vi "I_vs_Vw_V2w_V3w(V)_MFLI_PK_v4.0_measureR_phase.vi"() -> ()   [LabVIEW 2016]
uses:
  Labview Drivers/MFLI/LabOneLabVIEW-22.02.26577/LabOneLabVIEW-22.02.26577/Zurich Instruments LabOne/Public/Data/ziTypeDemodSampleSingle.ctl
  Labview Drivers/MFLI/LabOneLabVIEW-22.02.26577/LabOneLabVIEW-22.02.26577/Zurich Instruments LabOne/Public/Configure/ziSetValueDouble.vi
  Labview Drivers/MFLI/LabOneLabVIEW-22.02.26577/LabOneLabVIEW-22.02.26577/Zurich Instruments LabOne/Public/Configure/ziGetValueDemodSampleEx.vi
  Labview Drivers/MFLI/LabOneLabVIEW-22.02.26577/LabOneLabVIEW-22.02.26577/Zurich Instruments LabOne/Zurich Instruments LabOne.lvlib
panel:
  out "I2w vs Iw":cluster{dbl, "Field Reading":dbl}[](graph)=[{2.1337108522522826e-07, "Field Reading"=1.0007121497539348e-06}, {2.0018204953851064e-08, "Field Reading"=1.0969598663661376e-07}, {3.474074033482476e-08, "Field Reading"=1.9016075130631681e-07}, {5.6400419155691035e-08, "Field Reading"=2.706780203266455e-07}, {7.134741663483111e-08, "Field Reading"=3.625194153695155e-07}, {8.711957733763268e-08, "Field Reading"=4.6186456260881066e-07}, {1.039613386460647e-07, "Field Reading"=5.541771498802743e-07}, {1.290159481540569e-07, "Field Reading"=6.517488283090827e-07}, {1.442006622421336e-07, "Field Reading"=7.441421685111633e-07}, {1.6579779771841864e-07, "Field Reading"=8.4200282004452e-07}, {1.7667431320194624e-07, "Field Reading"=9.371894272094692e-07}, {2.0346799660082097e-07, "Field Reading"=1.0346819690568719e-06}, {2.1275449478314156e-07, "Field Reading"=1.1273455634288892e-06}, {2.2792303722372882e-07, "Field Reading"=1.2246113813938451e-06}, {2.506226161778463e-07, "Field Reading"=1.3169699353558023e-06}, {2.6686786096204173e-07, "Field Reading"=1.4106741902497636e-06}, {2.979630377408132e-07, "Field Reading"=1.5068897992871093e-06}, {3.1162936250255217e-07, "Field Reading"=1.6013785409354697e-06}, {3.2854904168138843e-07, "Field Reading"=1.7007967107121696e-06}, {3.4501678279448686e-07, "Field Reading"=1.7932741209540488e-06}, {3.5732655253185603e-07, "Field Reading"=1.891133061059139e-06}, {3.7678513716337806e-07, "Field Reading"=1.9837632139333797e-06}, {3.8857693765173823e-07, "Field Reading"=2.078638757139878e-06}, {4.070455630330932e-07, "Field Reading"=2.1777621608691614e-06}, {4.3651006057087547e-07, "Field Reading"=2.270487653250022e-06}, {4.535609885287045e-07, "Field Reading"=2.364817703267964e-06}, {4.800092323465329e-07, "Field Reading"=2.4630513126122318e-06}, {4.872172260420143e-07, "Field Reading"=2.560612214294704e-06}, {5.029105394973937e-07, "Field Reading"=2.653407522930296e-06}, {5.207137968885614e-07, "Field Reading"=2.7508846993110185e-06}, {5.449974912672081e-07, "Field Reading"=2.8437164663468094e-06}, {5.549097834910874e-07, "Field Reading"=2.941117576580943e-06}, {5.789147944756835e-07, "Field Reading"=3.0334756142859178e-06}, {5.940331669154695e-07, "Field Reading"=3.130923358288321e-06}, {6.192662248173834e-07, "Field Reading"=3.223457045619671e-06}, {6.338859460756282e-07, "Field Reading"=3.3210140787077685e-06}, {6.617730672082958e-07, "Field Reading"=3.4134337904467758e-06}, {6.708744764433933e-07, "Field Reading"=3.511218639909905e-06}, {6.876034184888421e-07, "Field Reading"=3.6064791588715936e-06}, {7.081705825683568e-07, "Field Reading"=3.704194984998823e-06}, {7.341349902267621e-07, "Field Reading"=3.796795088130521e-06}, {7.500412173627324e-07, "Field Reading"=3.894221622472711e-06}, {7.635282212201655e-07, "Field Reading"=3.986359362120525e-06}, {7.839559208505005e-07, "Field Reading"=4.084105589459172e-06}, {7.991337007295971e-07, "Field Reading"=4.176440151889332e-06}, {8.175550663233945e-07, "Field Reading"=4.274041338897146e-06}, {8.360511976155764e-07, "Field Reading"=4.366718612721536e-06}, {8.595654269642977e-07, "Field Reading"=4.46481586459238e-06}, {8.846044621269243e-07, "Field Reading"=4.559710869350914e-06}, {8.902214589762566e-07, "Field Reading"=4.6535858762473605e-06}, {9.13930972707384e-07, "Field Reading"=4.751211544539011e-06}, {9.218629476317926e-07, "Field Reading"=4.843674806906942e-06}, {9.389346568153207e-07, "Field Reading"=4.94148963023105e-06}, {9.661788530141893e-07, "Field Reading"=5.0340339305698605e-06}, {9.734275114489362e-07, "Field Reading"=5.134274890899915e-06}, {9.91273930192609e-07, "Field Reading"=5.227194198108034e-06}, {1.0062090937222443e-06, "Field Reading"=5.324543514118811e-06}, {1.0324830232331714e-06, "Field Reading"=5.417068558459935e-06}, {1.0500453704719826e-06, "Field Reading"=5.514414049876445e-06}, {1.0818020141498576e-06, "Field Reading"=5.606738838727315e-06}, {1.0919981214621985e-06, "Field Reading"=5.943499955969014e-06}, {1.1041062115858416e-06, "Field Reading"=5.802825671371831e-06}, {1.12928896400331e-06, "Field Reading"=5.8897635364887065e-06}, {1.1492595887607054e-06, "Field Reading"=5.986959246668246e-06}, {1.1525838773614565e-06, "Field Reading"=6.079112281920131e-06}, {1.1732006667255544e-06, "Field Reading"=6.176765549637453e-06}, {1.193444625294635e-06, "Field Reading"=6.2693583656248445e-06}, {1.2101538188023656e-06, "Field Reading"=6.369277338631168e-06}, {1.2318147585414787e-06, "Field Reading"=6.462177680852612e-06}, {1.2413491771177379e-06, "Field Reading"=6.554239754143973e-06}, {1.2731631837142253e-06, "Field Reading"=6.653541226069562e-06}, {1.2825564782833625e-06, "Field Reading"=6.7454110623267924e-06}, {1.2992348301055137e-06, "Field Reading"=6.843115368447837e-06}, {1.316693256967963e-06, "Field Reading"=6.935702965257668e-06}, {1.343852132299077e-06, "Field Reading"=7.033596304342718e-06}, {0.0003223256295561193, "Field Reading"=7.130369502789653e-06}, {0.0010682796466779994, "Field Reading"=7.237712618778445e-06}, {0.0011012721847992696, "Field Reading"=7.315133567183911e-06}, {0.0011336841810168491, "Field Reading"=7.4123545054478695e-06}, {0.0011614058556892847, "Field Reading"=7.504304430827025e-06}, {0.001182885890671154, "Field Reading"=7.602366955750201e-06}, {0.001200897535521615, "Field Reading"=7.69976061587441e-06}, {0.00121594401470624, "Field Reading"=7.792677109208386e-06}, {0.0012308027651267619, "Field Reading"=7.886128685028496e-06}, {0.0012456418637471253, "Field Reading"=7.983615236672288e-06}, {0.001257564969772003, "Field Reading"=8.075760842161778e-06}, {0.0012690336996615858, "Field Reading"=8.170723157183957e-06}, {0.0012814644345765262, "Field Reading"=8.268995175290895e-06}, {0.0012910253378675095, "Field Reading"=8.363131378141633e-06}, {0.001301444806581894, "Field Reading"=8.45644533427298e-06}, {0.0013106148752890106, "Field Reading"=8.551458283635111e-06}, {0.0013201336522581891, "Field Reading"=8.65161959339898e-06}, {0.0013282012490195363, "Field Reading"=8.74416723601607e-06}, {0.0013370451945670784, "Field Reading"=8.841765835802203e-06}, {0.001345475691336453, "Field Reading"=8.933978266213217e-06}, {0.0013541642420234728, "Field Reading"=9.031643266856203e-06}, {0.0013602243952778926, "Field Reading"=9.123705087732138e-06}, {0.0013678078924535615, "Field Reading"=9.221510724442928e-06}, {0.0013749931650039048, "Field Reading"=9.319154251910434e-06}, {0.0013817418853904447, "Field Reading"=9.409423170522308e-06}, {0.0013877620940512577, "Field Reading"=9.50720467327743e-06}, {0.0013893900209027232, "Field Reading"=9.522740574798281e-06}, {0.0013841293323999348, "Field Reading"=9.444358568387913e-06}, {0.0013770955503089543, "Field Reading"=9.34786117205707e-06}, {0.0013707463881856257, "Field Reading"=9.255459479065146e-06}, {0.0013638010752030354, "Field Reading"=9.157506360964617e-06}, {0.001356127430849226, "Field Reading"=9.065389480276688e-06}, {0.0013481807501391138, "Field Reading"=8.967105386552946e-06}, {0.0013407950243109453, "Field Reading"=8.872574329619889e-06}, {0.0013327879049762552, "Field Reading"=8.780745564878272e-06}, {0.0013239176518001648, "Field Reading"=8.686977265427215e-06}, {0.0013146578852826479, "Field Reading"=8.586299385882446e-06}, {0.0013048672888862206, "Field Reading"=8.493635331032656e-06}, {0.0012950842712132512, "Field Reading"=8.395823484571033e-06}, {0.0012855051336405129, "Field Reading"=8.303455420153361e-06}, {0.001274818349601112, "Field Reading"=8.209679742685101e-06}, {0.0012618971608759537, "Field Reading"=8.109946125115199e-06}, {0.0012494525821266837, "Field Reading"=8.017364894823338e-06}, {0.001235685913286103, "Field Reading"=7.919657723881713e-06}, {0.0012216877307261714, "Field Reading"=7.824897358413329e-06}, {0.0012037516065472435, "Field Reading"=7.727435253164315e-06}, {0.0011875344677767074, "Field Reading"=7.634970945479442e-06}, {0.0011690885694813937, "Field Reading"=7.537773175917453e-06}, {0.001143867923079635, "Field Reading"=7.445625913634191e-06}, {0.0011139726709101221, "Field Reading"=7.348337041113834e-06}, {0.0010813147907609588, "Field Reading"=7.255852572757193e-06}, {0.0008158901453383064, "Field Reading"=7.15654215348316e-06}, {0.00014586885402730632, "Field Reading"=7.065078532967033e-06}, {6.672313176192101e-06, "Field Reading"=6.97131792702715e-06}, {1.311378694927265e-06, "Field Reading"=6.8592321760864306e-06}, {1.318127585000335e-06, "Field Reading"=6.78165201436255e-06}, {1.2916070805813707e-06, "Field Reading"=6.684382236814962e-06}, {1.2637872492482735e-06, "Field Reading"=6.591615618281428e-06}, {1.2510857193087697e-06, "Field Reading"=6.49373019741343e-06}, {1.2409566576000475e-06, "Field Reading"=6.399307801408899e-06}, {1.215389141425889e-06, "Field Reading"=6.305912312991265e-06}, {1.1948309642776338e-06, "Field Reading"=6.211147873874382e-06}, {1.1729714746286896e-06, "Field Reading"=6.112674813622632e-06}, {1.1526746179431637e-06, "Field Reading"=6.015256707500007e-06}]
  in  "Number averaging":i32
  out "I2w_phase (deg)":dbl=40.57455732074348 format="%#_13g"
  out "Demod Sample Out 4":T1={"Timestamps (ticks)"=217071887690750, "X (Vrms)"=8.75456933556226e-07, "Y (Vrms)"=7.498226005787958e-07, "Osc Phase (deg)"=5.4774618983426535, "Freq (Hz)"=7.919000069023241, "DIO"=0, "AuxIn0 (V)"=-0.001673382503213361, "AuxIn1 (V)"=-0.0006673162570223212, "Trigger"=512}
  out "I2w (A)":dbl=1.1526746179431637e-06
  out "V2w_phase (deg)":dbl=40.57455732074348 format="%#_13g"
  out "Demod Sample Out 3":T1={"Timestamps (ticks)"=217071887690750, "X (Vrms)"=8.75456933556226e-07, "Y (Vrms)"=7.498226005787958e-07, "Osc Phase (deg)"=5.4774618983426535, "Freq (Hz)"=7.919000069023241, "DIO"=0, "AuxIn0 (V)"=-0.001673382503213361, "AuxIn1 (V)"=-0.0006673162570223212, "Trigger"=512}
  out "V2w (V)":dbl=1.1526746179431637e-06
  out "Iw_phase (deg)":dbl=-16.59997463839791 format="%#_13g"
  out "Vw_phase (deg)":dbl=40.57455732074348 format="%#_13g"
  out "Set Voltage(V)":dbl=4.384062043356605 format="%#_13g"
  out "Time(s)":dbl=185.322 format="%#_13g"
  out "Demod Sample Out 2":T1={"Timestamps (ticks)"=217071890701310, "X (Vrms)"=5.764492493379272e-06, "Y (Vrms)"=-1.7187028687058897e-06, "Osc Phase (deg)"=1.9746167692057917, "Freq (Hz)"=7.919000069023241, "DIO"=0, "AuxIn0 (V)"=-0.0006693530012853444, "AuxIn1 (V)"=0.0, "Trigger"=256}
  out "Demod Sample Out":T1={"Timestamps (ticks)"=217071887690750, "X (Vrms)"=8.75456933556226e-07, "Y (Vrms)"=7.498226005787958e-07, "Osc Phase (deg)"=5.4774618983426535, "Freq (Hz)"=7.919000069023241, "DIO"=0, "AuxIn0 (V)"=-0.001673382503213361, "AuxIn1 (V)"=-0.0006673162570223212, "Trigger"=512}
  in  "MFLI Current source/Voltage reader":string="DEV4496"
  out "Iw (A)":dbl=6.015256707500007e-06
  out "Vw (V)":dbl=1.1526746179431637e-06
  in  "Folder":path=path "D:/Heng/Nb3Br8_JJ/Sb.3_NBVJ01/20210115"
  in  "wait (ms) [Should be > TC]":u32=1000
  out "Iw vs Vw":cluster{dbl, "Field Reading":dbl}[](graph)=[{2.1337108522522826e-07, "Field Reading"=1.0007121497539348e-06}, {2.0018204953851064e-08, "Field Reading"=1.0969598663661376e-07}, {3.474074033482476e-08, "Field Reading"=1.9016075130631681e-07}, {5.6400419155691035e-08, "Field Reading"=2.706780203266455e-07}, {7.134741663483111e-08, "Field Reading"=3.625194153695155e-07}, {8.711957733763268e-08, "Field Reading"=4.6186456260881066e-07}, {1.039613386460647e-07, "Field Reading"=5.541771498802743e-07}, {1.290159481540569e-07, "Field Reading"=6.517488283090827e-07}, {1.442006622421336e-07, "Field Reading"=7.441421685111633e-07}, {1.6579779771841864e-07, "Field Reading"=8.4200282004452e-07}, {1.7667431320194624e-07, "Field Reading"=9.371894272094692e-07}, {2.0346799660082097e-07, "Field Reading"=1.0346819690568719e-06}, {2.1275449478314156e-07, "Field Reading"=1.1273455634288892e-06}, {2.2792303722372882e-07, "Field Reading"=1.2246113813938451e-06}, {2.506226161778463e-07, "Field Reading"=1.3169699353558023e-06}, {2.6686786096204173e-07, "Field Reading"=1.4106741902497636e-06}, {2.979630377408132e-07, "Field Reading"=1.5068897992871093e-06}, {3.1162936250255217e-07, "Field Reading"=1.6013785409354697e-06}, {3.2854904168138843e-07, "Field Reading"=1.7007967107121696e-06}, {3.4501678279448686e-07, "Field Reading"=1.7932741209540488e-06}, {3.5732655253185603e-07, "Field Reading"=1.891133061059139e-06}, {3.7678513716337806e-07, "Field Reading"=1.9837632139333797e-06}, {3.8857693765173823e-07, "Field Reading"=2.078638757139878e-06}, {4.070455630330932e-07, "Field Reading"=2.1777621608691614e-06}, {4.3651006057087547e-07, "Field Reading"=2.270487653250022e-06}, {4.535609885287045e-07, "Field Reading"=2.364817703267964e-06}, {4.800092323465329e-07, "Field Reading"=2.4630513126122318e-06}, {4.872172260420143e-07, "Field Reading"=2.560612214294704e-06}, {5.029105394973937e-07, "Field Reading"=2.653407522930296e-06}, {5.207137968885614e-07, "Field Reading"=2.7508846993110185e-06}, {5.449974912672081e-07, "Field Reading"=2.8437164663468094e-06}, {5.549097834910874e-07, "Field Reading"=2.941117576580943e-06}, {5.789147944756835e-07, "Field Reading"=3.0334756142859178e-06}, {5.940331669154695e-07, "Field Reading"=3.130923358288321e-06}, {6.192662248173834e-07, "Field Reading"=3.223457045619671e-06}, {6.338859460756282e-07, "Field Reading"=3.3210140787077685e-06}, {6.617730672082958e-07, "Field Reading"=3.4134337904467758e-06}, {6.708744764433933e-07, "Field Reading"=3.511218639909905e-06}, {6.876034184888421e-07, "Field Reading"=3.6064791588715936e-06}, {7.081705825683568e-07, "Field Reading"=3.704194984998823e-06}, {7.341349902267621e-07, "Field Reading"=3.796795088130521e-06}, {7.500412173627324e-07, "Field Reading"=3.894221622472711e-06}, {7.635282212201655e-07, "Field Reading"=3.986359362120525e-06}, {7.839559208505005e-07, "Field Reading"=4.084105589459172e-06}, {7.991337007295971e-07, "Field Reading"=4.176440151889332e-06}, {8.175550663233945e-07, "Field Reading"=4.274041338897146e-06}, {8.360511976155764e-07, "Field Reading"=4.366718612721536e-06}, {8.595654269642977e-07, "Field Reading"=4.46481586459238e-06}, {8.846044621269243e-07, "Field Reading"=4.559710869350914e-06}, {8.902214589762566e-07, "Field Reading"=4.6535858762473605e-06}, {9.13930972707384e-07, "Field Reading"=4.751211544539011e-06}, {9.218629476317926e-07, "Field Reading"=4.843674806906942e-06}, {9.389346568153207e-07, "Field Reading"=4.94148963023105e-06}, {9.661788530141893e-07, "Field Reading"=5.0340339305698605e-06}, {9.734275114489362e-07, "Field Reading"=5.134274890899915e-06}, {9.91273930192609e-07, "Field Reading"=5.227194198108034e-06}, {1.0062090937222443e-06, "Field Reading"=5.324543514118811e-06}, {1.0324830232331714e-06, "Field Reading"=5.417068558459935e-06}, {1.0500453704719826e-06, "Field Reading"=5.514414049876445e-06}, {1.0818020141498576e-06, "Field Reading"=5.606738838727315e-06}, {1.0919981214621985e-06, "Field Reading"=5.943499955969014e-06}, {1.1041062115858416e-06, "Field Reading"=5.802825671371831e-06}, {1.12928896400331e-06, "Field Reading"=5.8897635364887065e-06}, {1.1492595887607054e-06, "Field Reading"=5.986959246668246e-06}, {1.1525838773614565e-06, "Field Reading"=6.079112281920131e-06}, {1.1732006667255544e-06, "Field Reading"=6.176765549637453e-06}, {1.193444625294635e-06, "Field Reading"=6.2693583656248445e-06}, {1.2101538188023656e-06, "Field Reading"=6.369277338631168e-06}, {1.2318147585414787e-06, "Field Reading"=6.462177680852612e-06}, {1.2413491771177379e-06, "Field Reading"=6.554239754143973e-06}, {1.2731631837142253e-06, "Field Reading"=6.653541226069562e-06}, {1.2825564782833625e-06, "Field Reading"=6.7454110623267924e-06}, {1.2992348301055137e-06, "Field Reading"=6.843115368447837e-06}, {1.316693256967963e-06, "Field Reading"=6.935702965257668e-06}, {1.343852132299077e-06, "Field Reading"=7.033596304342718e-06}, {0.0003223256295561193, "Field Reading"=7.130369502789653e-06}, {0.0010682796466779994, "Field Reading"=7.237712618778445e-06}, {0.0011012721847992696, "Field Reading"=7.315133567183911e-06}, {0.0011336841810168491, "Field Reading"=7.4123545054478695e-06}, {0.0011614058556892847, "Field Reading"=7.504304430827025e-06}, {0.001182885890671154, "Field Reading"=7.602366955750201e-06}, {0.001200897535521615, "Field Reading"=7.69976061587441e-06}, {0.00121594401470624, "Field Reading"=7.792677109208386e-06}, {0.0012308027651267619, "Field Reading"=7.886128685028496e-06}, {0.0012456418637471253, "Field Reading"=7.983615236672288e-06}, {0.001257564969772003, "Field Reading"=8.075760842161778e-06}, {0.0012690336996615858, "Field Reading"=8.170723157183957e-06}, {0.0012814644345765262, "Field Reading"=8.268995175290895e-06}, {0.0012910253378675095, "Field Reading"=8.363131378141633e-06}, {0.001301444806581894, "Field Reading"=8.45644533427298e-06}, {0.0013106148752890106, "Field Reading"=8.551458283635111e-06}, {0.0013201336522581891, "Field Reading"=8.65161959339898e-06}, {0.0013282012490195363, "Field Reading"=8.74416723601607e-06}, {0.0013370451945670784, "Field Reading"=8.841765835802203e-06}, {0.001345475691336453, "Field Reading"=8.933978266213217e-06}, {0.0013541642420234728, "Field Reading"=9.031643266856203e-06}, {0.0013602243952778926, "Field Reading"=9.123705087732138e-06}, {0.0013678078924535615, "Field Reading"=9.221510724442928e-06}, {0.0013749931650039048, "Field Reading"=9.319154251910434e-06}, {0.0013817418853904447, "Field Reading"=9.409423170522308e-06}, {0.0013877620940512577, "Field Reading"=9.50720467327743e-06}, {0.0013893900209027232, "Field Reading"=9.522740574798281e-06}, {0.0013841293323999348, "Field Reading"=9.444358568387913e-06}, {0.0013770955503089543, "Field Reading"=9.34786117205707e-06}, {0.0013707463881856257, "Field Reading"=9.255459479065146e-06}, {0.0013638010752030354, "Field Reading"=9.157506360964617e-06}, {0.001356127430849226, "Field Reading"=9.065389480276688e-06}, {0.0013481807501391138, "Field Reading"=8.967105386552946e-06}, {0.0013407950243109453, "Field Reading"=8.872574329619889e-06}, {0.0013327879049762552, "Field Reading"=8.780745564878272e-06}, {0.0013239176518001648, "Field Reading"=8.686977265427215e-06}, {0.0013146578852826479, "Field Reading"=8.586299385882446e-06}, {0.0013048672888862206, "Field Reading"=8.493635331032656e-06}, {0.0012950842712132512, "Field Reading"=8.395823484571033e-06}, {0.0012855051336405129, "Field Reading"=8.303455420153361e-06}, {0.001274818349601112, "Field Reading"=8.209679742685101e-06}, {0.0012618971608759537, "Field Reading"=8.109946125115199e-06}, {0.0012494525821266837, "Field Reading"=8.017364894823338e-06}, {0.001235685913286103, "Field Reading"=7.919657723881713e-06}, {0.0012216877307261714, "Field Reading"=7.824897358413329e-06}, {0.0012037516065472435, "Field Reading"=7.727435253164315e-06}, {0.0011875344677767074, "Field Reading"=7.634970945479442e-06}, {0.0011690885694813937, "Field Reading"=7.537773175917453e-06}, {0.001143867923079635, "Field Reading"=7.445625913634191e-06}, {0.0011139726709101221, "Field Reading"=7.348337041113834e-06}, {0.0010813147907609588, "Field Reading"=7.255852572757193e-06}, {0.0008158901453383064, "Field Reading"=7.15654215348316e-06}, {0.00014586885402730632, "Field Reading"=7.065078532967033e-06}, {6.672313176192101e-06, "Field Reading"=6.97131792702715e-06}, {1.311378694927265e-06, "Field Reading"=6.8592321760864306e-06}, {1.318127585000335e-06, "Field Reading"=6.78165201436255e-06}, {1.2916070805813707e-06, "Field Reading"=6.684382236814962e-06}, {1.2637872492482735e-06, "Field Reading"=6.591615618281428e-06}, {1.2510857193087697e-06, "Field Reading"=6.49373019741343e-06}, {1.2409566576000475e-06, "Field Reading"=6.399307801408899e-06}, {1.215389141425889e-06, "Field Reading"=6.305912312991265e-06}, {1.1948309642776338e-06, "Field Reading"=6.211147873874382e-06}, {1.1729714746286896e-06, "Field Reading"=6.112674813622632e-06}, {1.1526746179431637e-06, "Field Reading"=6.015256707500007e-06}]
  out "data":dbl[](array[numeric])=[1.1526746179431637e-06, 6.015256707500007e-06, 3.1500000000000066, 184.117, 40.57455732074348, -16.59997463839791]
  in  "Step":dbl[](array[numeric])=[0.02, 0.02, 0.02] min=-3000.0 max=3000.0 format="%.1e"
  in  "To":dbl[](array[numeric])=[1.2, -1.2, 0.0] min=-3000.0 max=3000.0 format="%.1e"
  in  "From":dbl[](array[numeric])=[0.0, 1.2, -1.2] min=-3000.0 max=3000.0 format="%.1e"
  in  "file name":string="002_NBVJ01_IV(8mK)_I16_R34_ac(13.3337Hz)"
  out "File path":path=path "D:/Heng/Nb3Br8_JJ/Sb.3_NBVJ01/20210115/002_NBVJ01_IV(8mK)_I16_R34_ac(13.3337Hz).dat"
  # ".dat"
  # "Set MFLI Voltage output (V)"
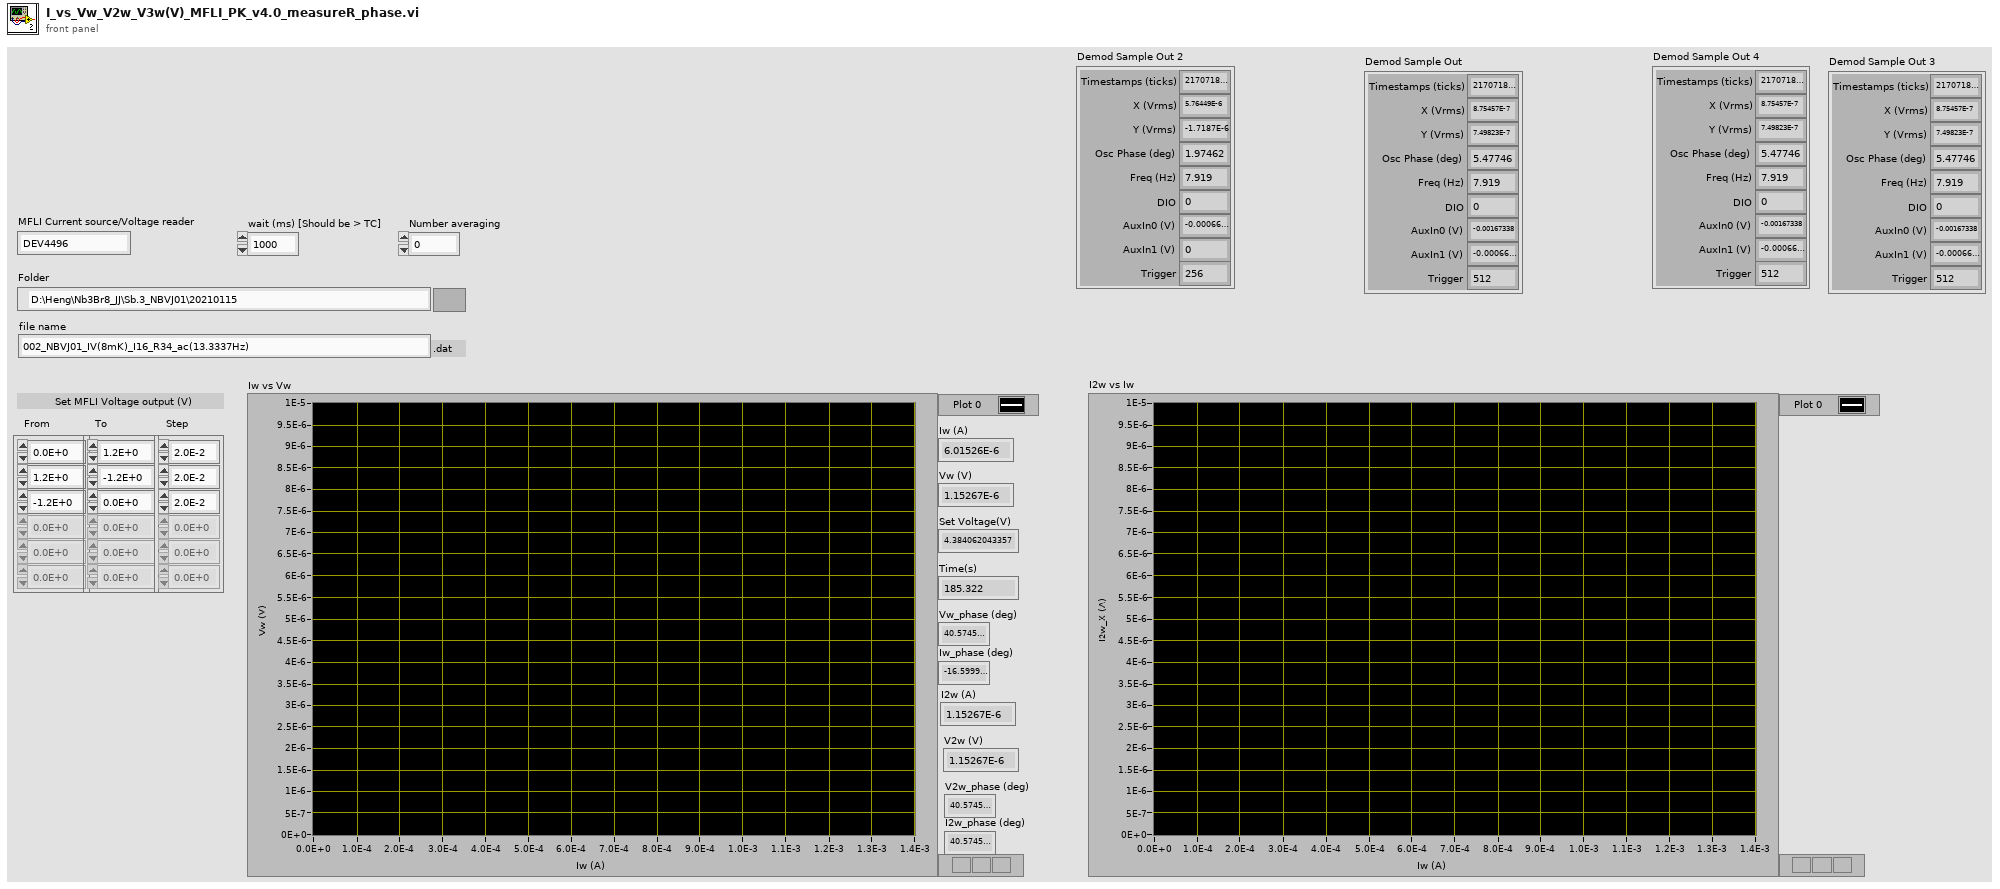
[diagram p1: front panel]
types:
  T1 = typedef "Zurich Instruments LabOne.lvlib/ziTypeDemodSampleSingle.ctl" = cluster{"Timestamps (ticks)":u64, "X (Vrms)":dbl, "Y (Vrms)":dbl, "Osc Phase (deg)":dbl, "Freq (Hz)":dbl, "DIO":u32, "AuxIn0 (V)":dbl, "AuxIn1 (V)":dbl, "Trigger":u32}
  T2 = enum16{"open", "replace", "create", "open or create", "replace or create", "replace or create with confirmation"}
  T3 = typedef "Zurich Instruments LabOne.lvlib/ziTypeHandle.ctl" = cluster{"handleValid":bool, "Conn":u64, "Path Prefix":string, "Handle":u64, "Connected":bool, "Clockbase(s)":dbl}
  T4 = cluster{"Average value":dbl, "Average value":dbl}
  T5 = cluster{"Average value":dbl, "Average value":dbl}[]
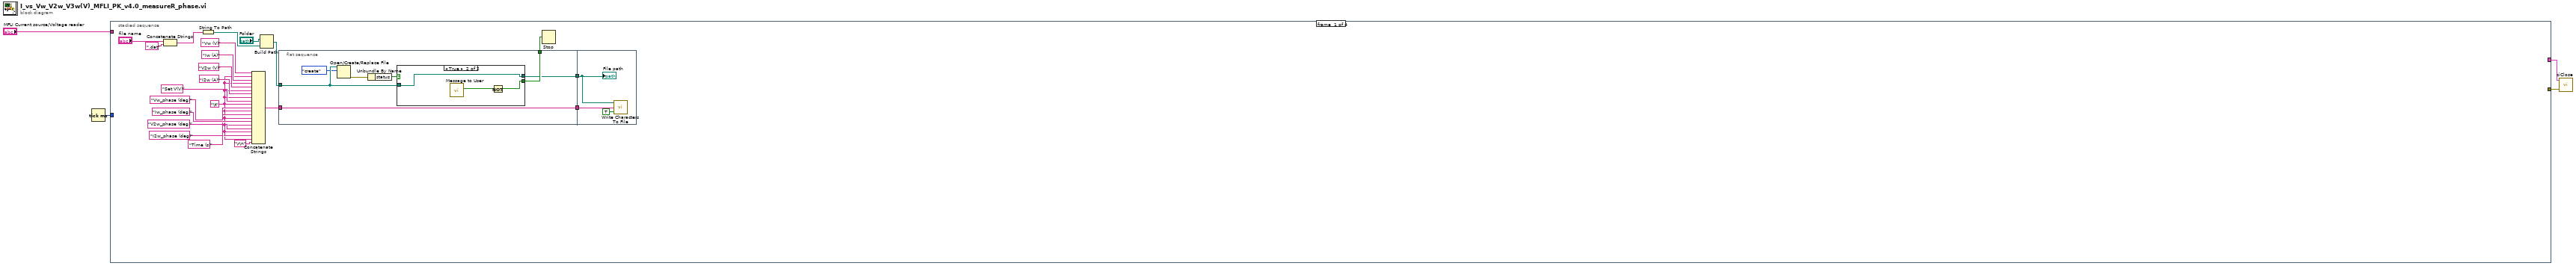
[diagram p0: block diagram]
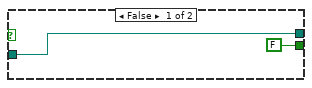
[diagram p2: hidden frame]
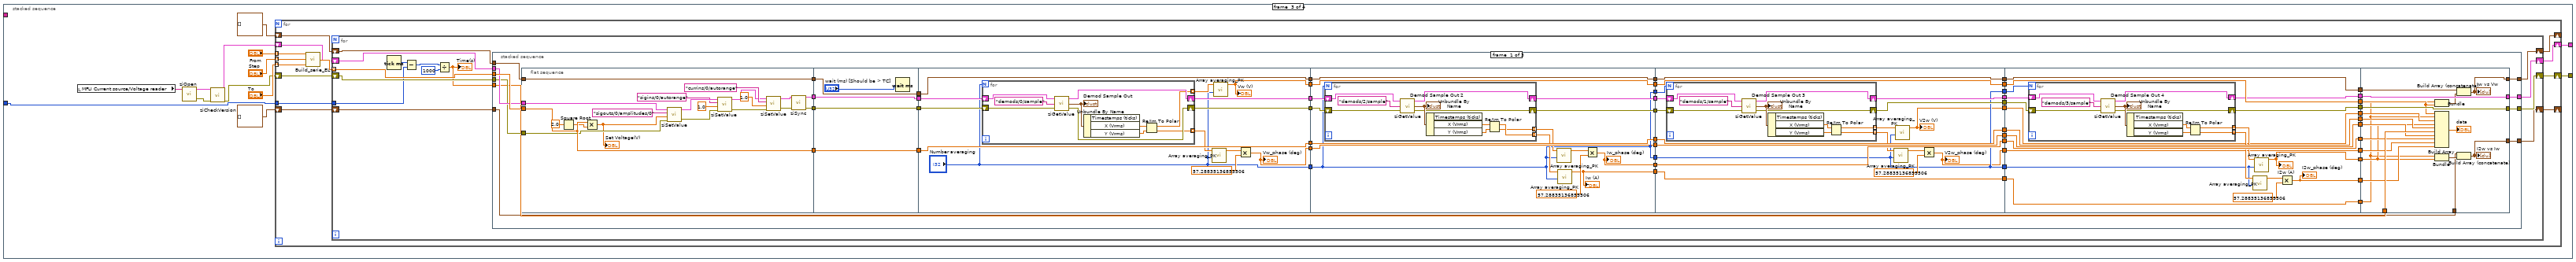
[diagram p4: hidden frame]
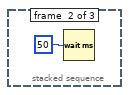
[diagram p5: hidden frame]
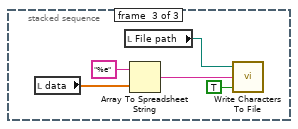
[diagram p6: hidden frame]
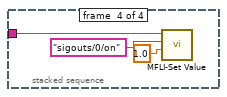
[diagram p7: hidden frame]
diagram:
  n1 = Tick Count (ms)() -> (millisecond timer value=w3:u32)
  n2 = stacked-sequence {
    tunnel: "MFLI Current source/Voltage reader" -> [_ _ _ w297]
    tunnel: w3 -> [_ _ w50 _]
    tunnel: [_ _ w48 _] -> w2
    tunnel: [_ _ w47 _] -> w1
    frame #0 {
      w5 = "\t"
      n3 = Concatenate Strings("file name", ".dat" ("string")) -> (w23:string)
      n4 = String To Path(string=w23) -> (path=w16:path)
      n5 = Concatenate Strings("Vw (V)" ("string"), w5, "Iw (A)" ("string"), w5, "V2w (V)" ("string"), w5, "I2w (A)" ("string"), w5, "Set V(V)" ("string"), w5, "Time (s)", w5, "Vw_phase (deg)", w5, "Iw_phase (deg)", w5, "V2w_phase (deg)", w5, "I2w_phase (deg)", w5, "\r\n") -> (w24:string)
      n6 = Build Path(base path="Folder", name or relative path=w16) -> (appended path=w15:path)
      n7 = flat-sequence {
        tunnel: w15 -> [w30]
        tunnel: w24 -> [w33]
        tunnel: [w33] -> w26
        tunnel: [w32] -> w21
        tunnel: [w31] -> w25
        tunnel: w26 -> [w40]
        tunnel: w25 -> [w39]
        frame #0 {
          n8 = Open/Create/Replace File(file path (use dialog)=w30, operation (0:open)=T2."create") -> (error out=w29:errorcluster)  [unwired: 4 in, 2 out]
          n9 = Unbundle By Name(w29) -> ("status"=w27:bool)
          n10 = case shown="True" w27 {
            tunnel: [FALSE ("Yes") w37] -> w32
            tunnel: [w34 w36] -> w31
            tunnel: w30 -> [w34 w36]
            frame False {
            }
            frame True {
              n11 = call "Message to User"() -> ("Yes"=w38:bool)  [unwired: 10 in, 1 out]
              n12 = Not(x=w38) -> (.not. x?=w37:bool)
            }
          }
        }
        frame #1 {
          n13 = call <vilib>:"Write Characters To File.vi"("append to file? (new file:F)"=TRUE, "character string"=w40, "file path (dialog if empty)"=w39) -> ()  [unwired: 2 in, 1 out]
          "File path" <- w39
        }
      }
      n14 = Stop(stop? (T)=w21) -> ()
    }
    frame #1 {
    }
    frame #2 {
      n15 = local read "MFLI Current source/Voltage reader"() -> (w44:string)
      n16 = call "ziOpen.vi"("Address"=w44) -> ("Error Out"=w45:errorcluster, "HandleOut"=w46:T3)  [unwired: 3 in, 1 out]
      n17 = call "ziCheckVersion.vi"("Handle In"=w46, "Error In"=w45) -> ("Handle Out"=w43:T3, "Error Out"=w42:errorcluster)  [unwired: 11 in, 1 out]
      n18 = for {
        tunnel: "From" -> [w64] mode=indexing
        tunnel: "To" -> [w63] mode=indexing
        tunnel: "Step" -> [w62] mode=indexing
        shift-right: [w66] -> _
        shift-left: cluster{dbl, "Field Reading":dbl}[] [] -> [w67]
        tunnel: w50 -> [w61]
        shift-right: [w60] -> _
        shift-left: cluster{dbl, "Field Reading":dbl}[] [] -> [w59]
        shift-right: [w58] -> w48
        shift-left: w43 -> [w56]
        shift-right: [w57] -> w47
        shift-left: w42 -> [w55]
        n19 = call "Build_serie_EL.vi"("end value"=w63, "increment"=w62, "start value"=w64) -> ("output array"=w65:dbl[])
        n20 = for {
          tunnel: w65 -> [w81] mode=indexing
          shift-right: [w79] -> w66
          shift-left: w67 -> [w80]
          shift-right: [w76] -> w58
          shift-left: w56 -> [w78]
          shift-right: [w75] -> w57
          shift-left: w55 -> [w77]
          tunnel: w61 -> [w71]
          shift-right: [w69] -> w60
          shift-left: w59 -> [w68]
          n21 = Tick Count (ms)() -> (millisecond timer value=w72:u32)
          n22 = Subtract(x=w72, y=w71) -> (x-y=w73:u32)
          n23 = Divide(x=w73, y=1000) -> (x/y=w70:dbl)
          "Time(s)" <- w70
          n24 = stacked-sequence {
            tunnel: w81 -> [w138 _ _]
            tunnel: w80 -> [w139 _ _]
            tunnel: [w140 _ _] -> w79
            tunnel: w78 -> [w129 _ _]
            tunnel: w77 -> [w128 _ _]
            tunnel: [w122 _ _] -> w76
            tunnel: [w121 _ _] -> w75
            tunnel: w70 -> [w120 _ _]
            tunnel: [w83 _ _] -> w69
            tunnel: w68 -> [w82 _ _]
            frame #0 {
              n25 = flat-sequence {
                tunnel: [w160] -> w135
                tunnel: [w159] -> w134
                tunnel: w138 -> [w159]
                tunnel: w139 -> [w160]
                tunnel: [w142] -> w131
                tunnel: [w143] -> w130
                tunnel: w129 -> [w145]
                tunnel: w128 -> [w144]
                tunnel: w135 -> [w165]
                tunnel: [w165] -> w137
                tunnel: w134 -> [w164]
                tunnel: [w164] -> w136
                tunnel: [w162] -> w133
                tunnel: [w161] -> w132
                tunnel: w131 -> [w161]
                tunnel: w130 -> [w162]
                tunnel: [w170] -> w127
                tunnel: [w178] -> w126
                tunnel: [w177] -> w125
                tunnel: w132 -> [w176]
                tunnel: w133 -> [w175]
                tunnel: w137 -> [w178]
                tunnel: w136 -> [w177]
                tunnel: [w174] -> w124
                tunnel: [w173] -> w123
                tunnel: [w172] -> w119
                tunnel: ["Number averaging"] -> w96
                tunnel: w127 -> [w197]
                tunnel: [w197] -> w118
                tunnel: w126 -> [w203]
                tunnel: [w203] -> w117
                tunnel: w125 -> [w202]
                tunnel: [w202] -> w116
                tunnel: w124 -> [w201]
                tunnel: w123 -> [w200]
                tunnel: [w199] -> w115
                tunnel: [w198] -> w114
                tunnel: [w193] -> w113
                tunnel: [w194] -> w112
                tunnel: w119 -> [w196]
                tunnel: [w196] -> w111
                tunnel: w96 -> [w189]
                tunnel: [w189] -> w94
                tunnel: [w189] -> w93
                tunnel: w118 -> [w231]
                tunnel: [w231] -> w110
                tunnel: w117 -> [w230]
                tunnel: [w230] -> w108
                tunnel: w116 -> [w229]
                tunnel: [w229] -> w106
                tunnel: w115 -> [w224]
                tunnel: w114 -> [w223]
                tunnel: [w218] -> w104
                tunnel: w113 -> [w228]
                tunnel: [w228] -> w102
                tunnel: w112 -> [w227]
                tunnel: [w227] -> w100
                tunnel: w111 -> [w226]
                tunnel: [w226] -> w98
                tunnel: [w219] -> w95
                tunnel: w94 -> [w217]
                tunnel: w93 -> [w216]
                tunnel: [w216] -> w91
                tunnel: [w216] -> w90
                tunnel: [w215] -> w88
                tunnel: [w214] -> w85
                tunnel: w110 -> [w261]
                tunnel: [w261] -> w109
                tunnel: w108 -> [w260]
                tunnel: [w260] -> w107
                tunnel: w106 -> [w259]
                tunnel: [w259] -> w105
                tunnel: w104 -> [w253]
                tunnel: [w251] -> w103
                tunnel: w102 -> [w258]
                tunnel: [w258] -> w101
                tunnel: w100 -> [w257]
                tunnel: [w257] -> w99
                tunnel: w98 -> [w256]
                tunnel: [w256] -> w97
                tunnel: w95 -> [w254]
                tunnel: [w252] -> w92
                tunnel: w91 -> [w247]
                tunnel: w90 -> [w246]
                tunnel: [w245] -> w89
                tunnel: w88 -> [w244]
                tunnel: [w244] -> w87
                tunnel: [w243] -> w86
                tunnel: w85 -> [w242]
                tunnel: [w242] -> w84
                tunnel: w109 -> [w274]
                tunnel: [w289] -> w140
                tunnel: w107 -> [w288]
                tunnel: w105 -> [w276]
                tunnel: [w287] -> w122
                tunnel: [w286] -> w121
                tunnel: w103 -> [w286]
                tunnel: w101 -> [w273]
                tunnel: w120 -> [w284]
                tunnel: w99 -> [w283]
                tunnel: w97 -> [w282]
                tunnel: w92 -> [w287]
                tunnel: w89 -> [w275]
                tunnel: w87 -> [w281]
                tunnel: w86 -> [w280]
                tunnel: w84 -> [w279]
                tunnel: [w277] -> w83
                tunnel: w82 -> [w272]
                frame #0 {
                  n26 = Square Root(x=2.0) -> (sqrt(x)=w158:dbl)
                  n27 = Multiply(x=w159, y=w158) -> (x*y=w141:dbl)
                  "Set Voltage(V)" <- w141
                  n28 = call-poly "ziSetValue.vi"("Error In"=w144, "Value"=w141, "Path"="sigouts/0/amplitudes/0", "Handle In"=w145) -> ("Error Out"=w152:errorcluster, "Handle Out"=w155:T3)  [unwired: 1 in]
                  n29 = call-poly "ziSetValue.vi"("Error In"=w152, "Value"=1.0, "Path"="sigins/0/autorange", "Handle In"=w155) -> ("Error Out"=w148:errorcluster, "Handle Out"=w149:T3)  [unwired: 1 in]
                  n30 = call-poly "ziSetValue.vi"("Error In"=w148, "Value"=1.0, "Path"="currins/0/autorange", "Handle In"=w149) -> ("Error Out"=w146:errorcluster, "Handle Out"=w147:T3)  [unwired: 1 in]
                  n31 = call "ziSync.vi"("Handle In"=w147, "Error In"=w146) -> ("Handle Out"=w143:T3, "Error Out"=w142:errorcluster)  [unwired: 12 in]
                }
                frame #1 {
                  n32 = Wait (ms)(milliseconds to wait="wait (ms) [Should be > TC]") -> ()  [unwired: 1 out]
                }
                frame #2 {
                  n33 = for {
                    N: "Number averaging" -> [_]
                    tunnel: [w180] -> w169 mode=indexing
                    tunnel: [w179] -> w167 mode=indexing
                    shift-right: [w183] -> w173
                    shift-left: w176 -> [w186]
                    shift-right: [w184] -> w174
                    shift-left: w175 -> [w185]
                    n34 = call-poly "ziGetValue.vi"("error in"=w186, "Path"="demods/0/sample", "Handle In"=w185) -> ("error out"=w183:errorcluster, "Demod Sample Out"=w187:T1, "Handle Out"=w184:T3)
                    "Demod Sample Out" <- w187
                    n35 = Unbundle By Name(w187) -> ("X (Vrms)"=w182:dbl, "Y (Vrms)"=w181:dbl)  [unwired: 1 out]
                    n36 = Re/Im To Polar(2:w181, 3:w182) -> (0:w179:dbl, 1:w180:dbl)
                  }
                  n37 = call "Array averaging_PK.vi"("Number averaging"="Number averaging", "numeric array"=w167) -> ("Average value"=w168:dbl)  [unwired: 9 in]
                  n38 = call "Array averaging_PK.vi"("Number averaging"="Number averaging", "numeric array"=w169) -> ("Average value"=w170:dbl)  [unwired: 9 in]
                  "Vw (V)" <- w170
                  n39 = Multiply(x=w168, y=57.28835136855506) -> (x*y=w172:dbl)
                  "Vw_phase (deg)" <- w172
                }
                frame #3 {
                  n40 = for {
                    N: w189 -> [_]
                    tunnel: [w205] -> w191 mode=indexing
                    tunnel: [w204] -> w190 mode=indexing
                    shift-right: [w209] -> w199
                    shift-left: w201 -> [w211]
                    shift-right: [w208] -> w198
                    shift-left: w200 -> [w210]
                    n41 = call-poly "ziGetValue.vi"("error in"=w210, "Path"="demods/2/sample", "Handle In"=w211) -> ("error out"=w208:errorcluster, "Demod Sample Out"=w212:T1, "Handle Out"=w209:T3)
                    "Demod Sample Out 2" <- w212
                    n42 = Unbundle By Name(w212) -> ("X (Vrms)"=w206:dbl, "Y (Vrms)"=w207:dbl)  [unwired: 1 out]
                    n43 = Re/Im To Polar(2:w207, 3:w206) -> (0:w204:dbl, 1:w205:dbl)
                  }
                  n44 = call "Array averaging_PK.vi"("Number averaging"=w189, "numeric array"=w190) -> ("Average value"=w192:dbl)  [unwired: 9 in]
                  n45 = call "Array averaging_PK.vi"("Number averaging"=w189, "numeric array"=w191) -> ("Average value"=w193:dbl)  [unwired: 9 in]
                  "Iw (A)" <- w193
                  n46 = Multiply(x=w192, y=57.28835136855506) -> (x*y=w194:dbl)
                  "Iw_phase (deg)" <- w194
                }
                frame #4 {
                  n47 = for {
                    N: w217 -> [_]
                    tunnel: [w237] -> w220 mode=indexing
                    tunnel: [w236] -> w222 mode=indexing
                    shift-right: [w233] -> w219
                    shift-left: w224 -> [w235]
                    shift-right: [w232] -> w218
                    shift-left: w223 -> [w234]
                    n48 = call-poly "ziGetValue.vi"("error in"=w234, "Path"="demods/1/sample", "Handle In"=w235) -> ("error out"=w232:errorcluster, "Demod Sample Out"=w240:T1, "Handle Out"=w233:T3)
                    "Demod Sample Out 3" <- w240
                    n49 = Unbundle By Name(w240) -> ("X (Vrms)"=w239:dbl, "Y (Vrms)"=w238:dbl)  [unwired: 1 out]
                    n50 = Re/Im To Polar(2:w238, 3:w239) -> (0:w236:dbl, 1:w237:dbl)
                  }
                  n51 = call "Array averaging_PK.vi"("Number averaging"=w216, "numeric array"=w222) -> ("Average value"=w221:dbl)  [unwired: 9 in]
                  n52 = call "Array averaging_PK.vi"("Number averaging"=w216, "numeric array"=w220) -> ("Average value"=w215:dbl)  [unwired: 9 in]
                  "V2w (V)" <- w215
                  n53 = Multiply(x=w221, y=57.28835136855506) -> (x*y=w214:dbl)
                  "V2w_phase (deg)" <- w214
                }
                frame #5 {
                  n54 = for {
                    N: w247 -> [_]
                    tunnel: [w267] -> w250 mode=indexing
                    tunnel: [w266] -> w248 mode=indexing
                    shift-right: [w263] -> w252
                    shift-left: w254 -> [w265]
                    shift-right: [w262] -> w251
                    shift-left: w253 -> [w264]
                    n55 = call-poly "ziGetValue.vi"("error in"=w264, "Path"="demods/3/sample", "Handle In"=w265) -> ("error out"=w262:errorcluster, "Demod Sample Out"=w270:T1, "Handle Out"=w263:T3)
                    "Demod Sample Out 4" <- w270
                    n56 = Unbundle By Name(w270) -> ("X (Vrms)"=w269:dbl, "Y (Vrms)"=w268:dbl)  [unwired: 1 out]
                    n57 = Re/Im To Polar(2:w268, 3:w269) -> (0:w266:dbl, 1:w267:dbl)
                  }
                  n58 = call "Array averaging_PK.vi"("Number averaging"=w246, "numeric array"=w248) -> ("Average value"=w249:dbl)  [unwired: 9 in]
                  n59 = call "Array averaging_PK.vi"("Number averaging"=w246, "numeric array"=w250) -> ("Average value"=w245:dbl)  [unwired: 9 in]
                  "I2w (A)" <- w245
                  n60 = Multiply(x=w249, y=57.28835136855506) -> (x*y=w243:dbl)
                  "I2w_phase (deg)" <- w243
                }
                frame #6 {
                  n61 = Bundle("Average value"=w273, "Average value"=w274) -> (w285:T4)  [unwired: 1 in]
                  n62 = Build Array(w274, w273, w281, w275, w276, w284, w282, w283, w279, w280) -> (→"data":dbl[])
                  n63 = Bundle("Average value"=w273, "Average value"=w275) -> (w278:T4)  [unwired: 1 in]
                  n64 = Build Array (concatenate)(w288, w285) -> (w289:T5)
                  "Iw vs Vw" <- w289
                  n65 = Build Array (concatenate)(w272, w278) -> (w277:T5)
                  "I2w vs Iw" <- w277
                }
              }
            }
            frame #1 {
              n66 = Wait (ms)(milliseconds to wait=u32 50) -> ()  [unwired: 1 out]
            }
            frame #2 {
              n67 = local read "data"() -> (w292:dbl[])
              n68 = local read "File path"() -> (w294:path)
              n69 = Array To Spreadsheet String(array=w292, 3:"%e" ("format string")) -> (spreadsheet string=w295:string)  [unwired: 1 in]
              n70 = call <vilib>:"Write Characters To File.vi"("append to file? (new file:F)"=TRUE, "character string"=w295, "file path (dialog if empty)"=w294) -> ()  [unwired: 2 in, 1 out]
            }
          }
        }
      }
    }
    frame #3 {
      n71 = call "MFLI-Set Value.vi"("Value"=1.0, "Path"="sigouts/0/on", "MFLI Current source/Voltage reader"=w297) -> ()  [unwired: 9 in]
    }
  }
  n72 = call "ziClose.vi"("Error In"=w1, "Handle In"=w2) -> ()  [unwired: 4 out]
